vi "Remove Children.vi"(8 "error in (no error)":errorcluster, 11 "Element Array in":refnum<class "Element Array.lvclass">) -> (0 "error out":errorcluster, 3 "Element Array out":refnum<class "Element Array.lvclass">)   [LabVIEW 2020, in "VILab.lvlib" / "Element Array.lvclass"]
uses:
  Element Array.lvclass
  Attribute/Attribute.lvclass
  Element Array.lvclass/Element Array.ctl
  Data Item/Data Item.lvclass
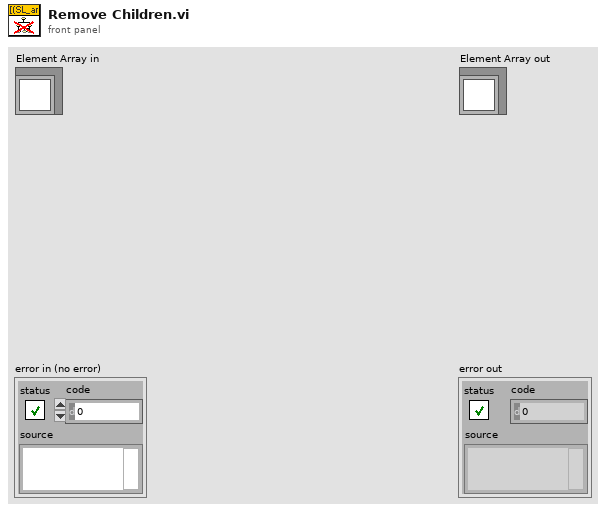
[diagram p1: front panel]
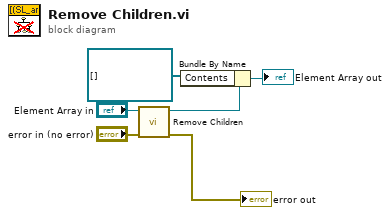
[diagram p0: block diagram]
diagram:
  n1 = call-parent "Remove Children.vi"("error in (no error)"="error in (no error)", "Data Item in"="Element Array in") -> ("error out"=→"error out":errorcluster, "Data Item out"=w3:refnum<class "Element Array.lvclass">)  [unwired: 8 in]
  n2 = Bundle By Name(cluster=w3, "Contents"=refnum<class "Attribute.lvclass">[] []) -> (→"Element Array out":refnum<class "Element Array.lvclass">)
